vi "Emballage_BDD_GVF_softSAFE.vi"(2 "Error in":errorcluster caption="Error in (no error)", 3 "Énum":enum16{"SET", "GET"}(ring), 4 "SOFTSAFE":bool) -> (0 "Error out":errorcluster, 1 "SOFTSAFE":bool)   [LabVIEW 2020]
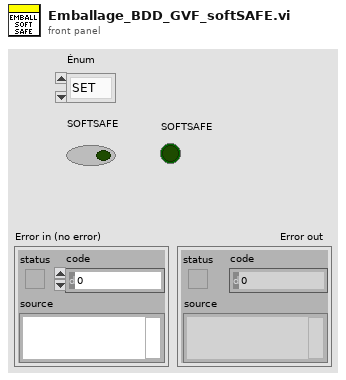
[diagram p1: front panel]
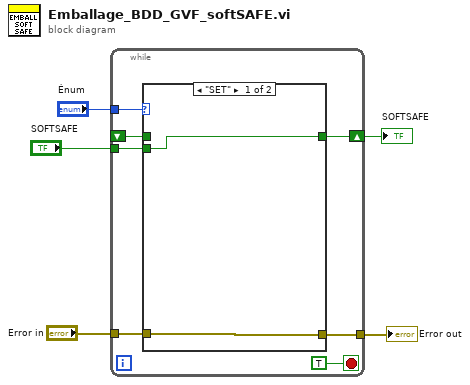
[diagram p0: block diagram]
diagram:
  n1 = while {
    tunnel: "Énum" -> [w12]
    shift-right: [w11] -> w3
    shift-left: _ -> [w9]
    tunnel: "SOFTSAFE" -> [w10]
    tunnel: "Error in" -> [w7]
    tunnel: [w6] -> w1
    stop <- TRUE stop-if-true
    n2 = case shown="\"SET\"" w12 {
      tunnel: [w14 w16] -> w11
      tunnel: w10 -> [w14 _]
      tunnel: w9 -> [_ w16]
      tunnel: w7 -> [w13 w15]
      tunnel: [w13 w15] -> w6
      frame "SET" {
      }
      frame "GET", Default {
      }
    }
  }
  "SOFTSAFE" <- w3
  "Error out" <- w1
